vi "PumpValveHeater2.vi"() -> ()   [LabVIEW 2015]
uses:
  PumpValve.ctl
  <vilib>/DAQmx/read.llb/DAQmx Read (Analog 1D Wfm NChan 1Samp).vi
  <vilib>/DAQmx/write.llb/DAQmx Write (Digital 1D Bool NChan 1Samp 1Line).vi
  <vilib>/DAQmx/miscellaneous.llb/DAQmx Fill In Error Info.vi
  <vilib>/addons/control/pid/pid.llb/PID (DBL).vi
  <vilib>/addons/control/pid/pid.llb/PID Advanced (DBL).vi
  <vilib>/addons/control/pid/NI_PID_pid.lvlib
panel:
  out "Temp Chart 2":waveform(dbl)(graph)
  out "Pressure (mBar) 2":dbl format="%#_13g"
  out "Voltage Reading (Pressure)":dbl format="%#_13g"
  out "Pressure Chart":waveform(dbl)(graph)
  in  "stop":bool
  out "Voltage Reading(Temp)":dbl format="%#_13g"
  out "Temperature (Celcius)":dbl format="%#.1g"
  out "Temp(C)":dbl(slide) scale=-10.0..100.0
  out "Temp Chart":waveform(dbl)(graph)
  out "Duty Cycle from Control Value":dbl
  out "Numeric":dbl
  out "Heater On/off":bool
  out "Control Value (Temp Sensor)":dbl(knob) scale=0.0..100.0
  in  "Stop Maintaining Temp":bool
  in  "PID gains Temp":T1={"proportional gain (Kc)"=1.0, "integral time (Ti, min)"=0.01, "derivative time (Td, min)"=0.0} {"derivative time (Td, min)" format="%.3f"; "integral time (Ti, min)" format="%.3f"; "proportional gain (Kc)" format="%.3f"}
  in  "Temp Setting":dbl
  in  "Maintain Temp":bool
  in  "Stop Maintaining Pressure":bool
  in  "PID gains":T1={"proportional gain (Kc)"=1.0, "integral time (Ti, min)"=0.01, "derivative time (Td, min)"=0.0} {"derivative time (Td, min)" format="%.3f"; "integral time (Ti, min)" format="%.3f"; "proportional gain (Kc)" format="%.3f"}
  out "Meter (Pressure Sensor)":dbl(knob) scale=0.0..10.0
  in  "Pressure Setting":dbl
  in  "Maintain pressure":bool
  in  "On/Off Temp":bool
  in  "Manual Mode Temp":bool
  in  "stop controller":bool
  in  "Duty cycle % (0-100) (manual only)":dbl=50.0
  in  "stop PWM":bool
  in  "Steps in a cycle":i32=256
  in  "Cycle time (s)":dbl=5.0
  in  "On/Off (Pump)":bool
  in  "Open/Close (Blue)":bool
  in  "Open/Close (Green)":bool
  in  "Manual Mode Pump/Valve":bool
  out "Invalid fill%":bool
  out "Tank":u32(slide) scale=0.0..100.0
  in  "Drain %":u32
  in  "Fill %":u32
  in  "Drain":bool
  in  "Stop Program":bool
  in  "Fill":bool
  # "Temp only adjusts up (do nothing to cool?)"
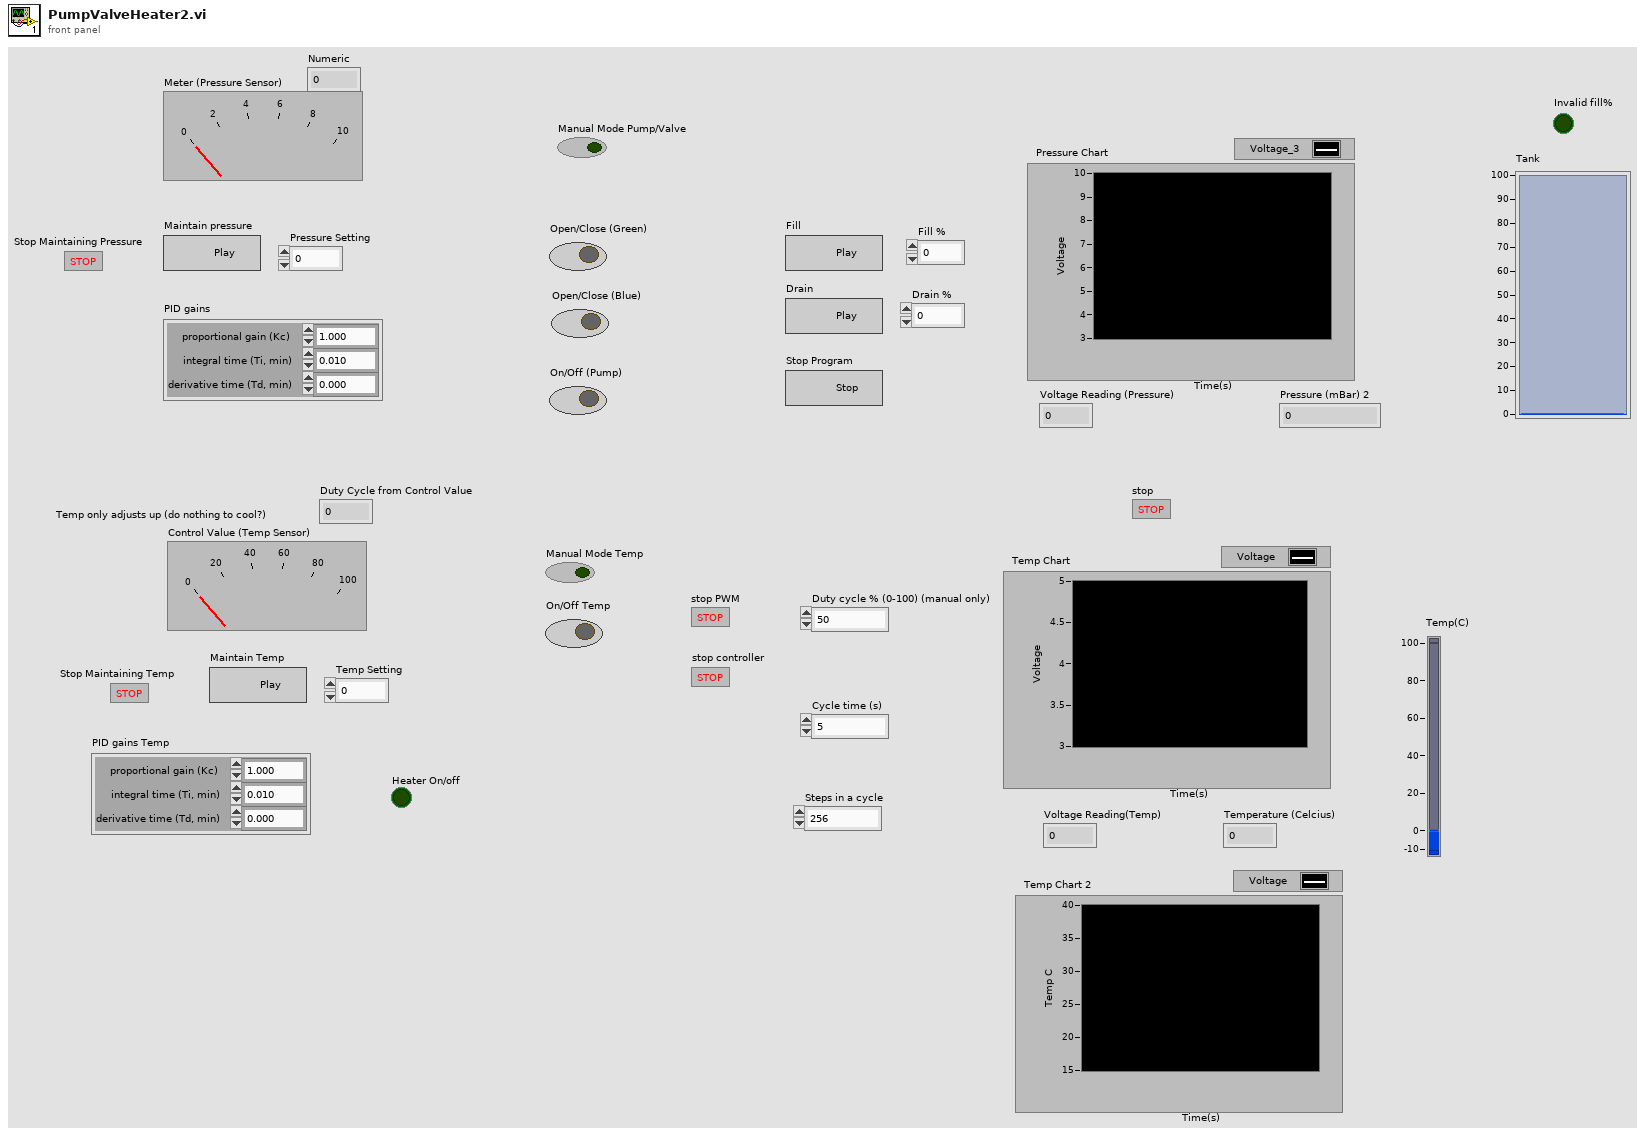
[diagram p1: front panel]
types:
  T1 = cluster{"proportional gain (Kc)":dbl, "integral time (Ti, min)":dbl, "derivative time (Td, min)":dbl}
  T2 = typedef "PumpValve.ctl" = enum16{"PressureSetting", "ManualPressure", "ManualTemp", "Idle Temp", "Set Temp", "Initialize", "Idle", "Fill", "Drain", "Stop"}
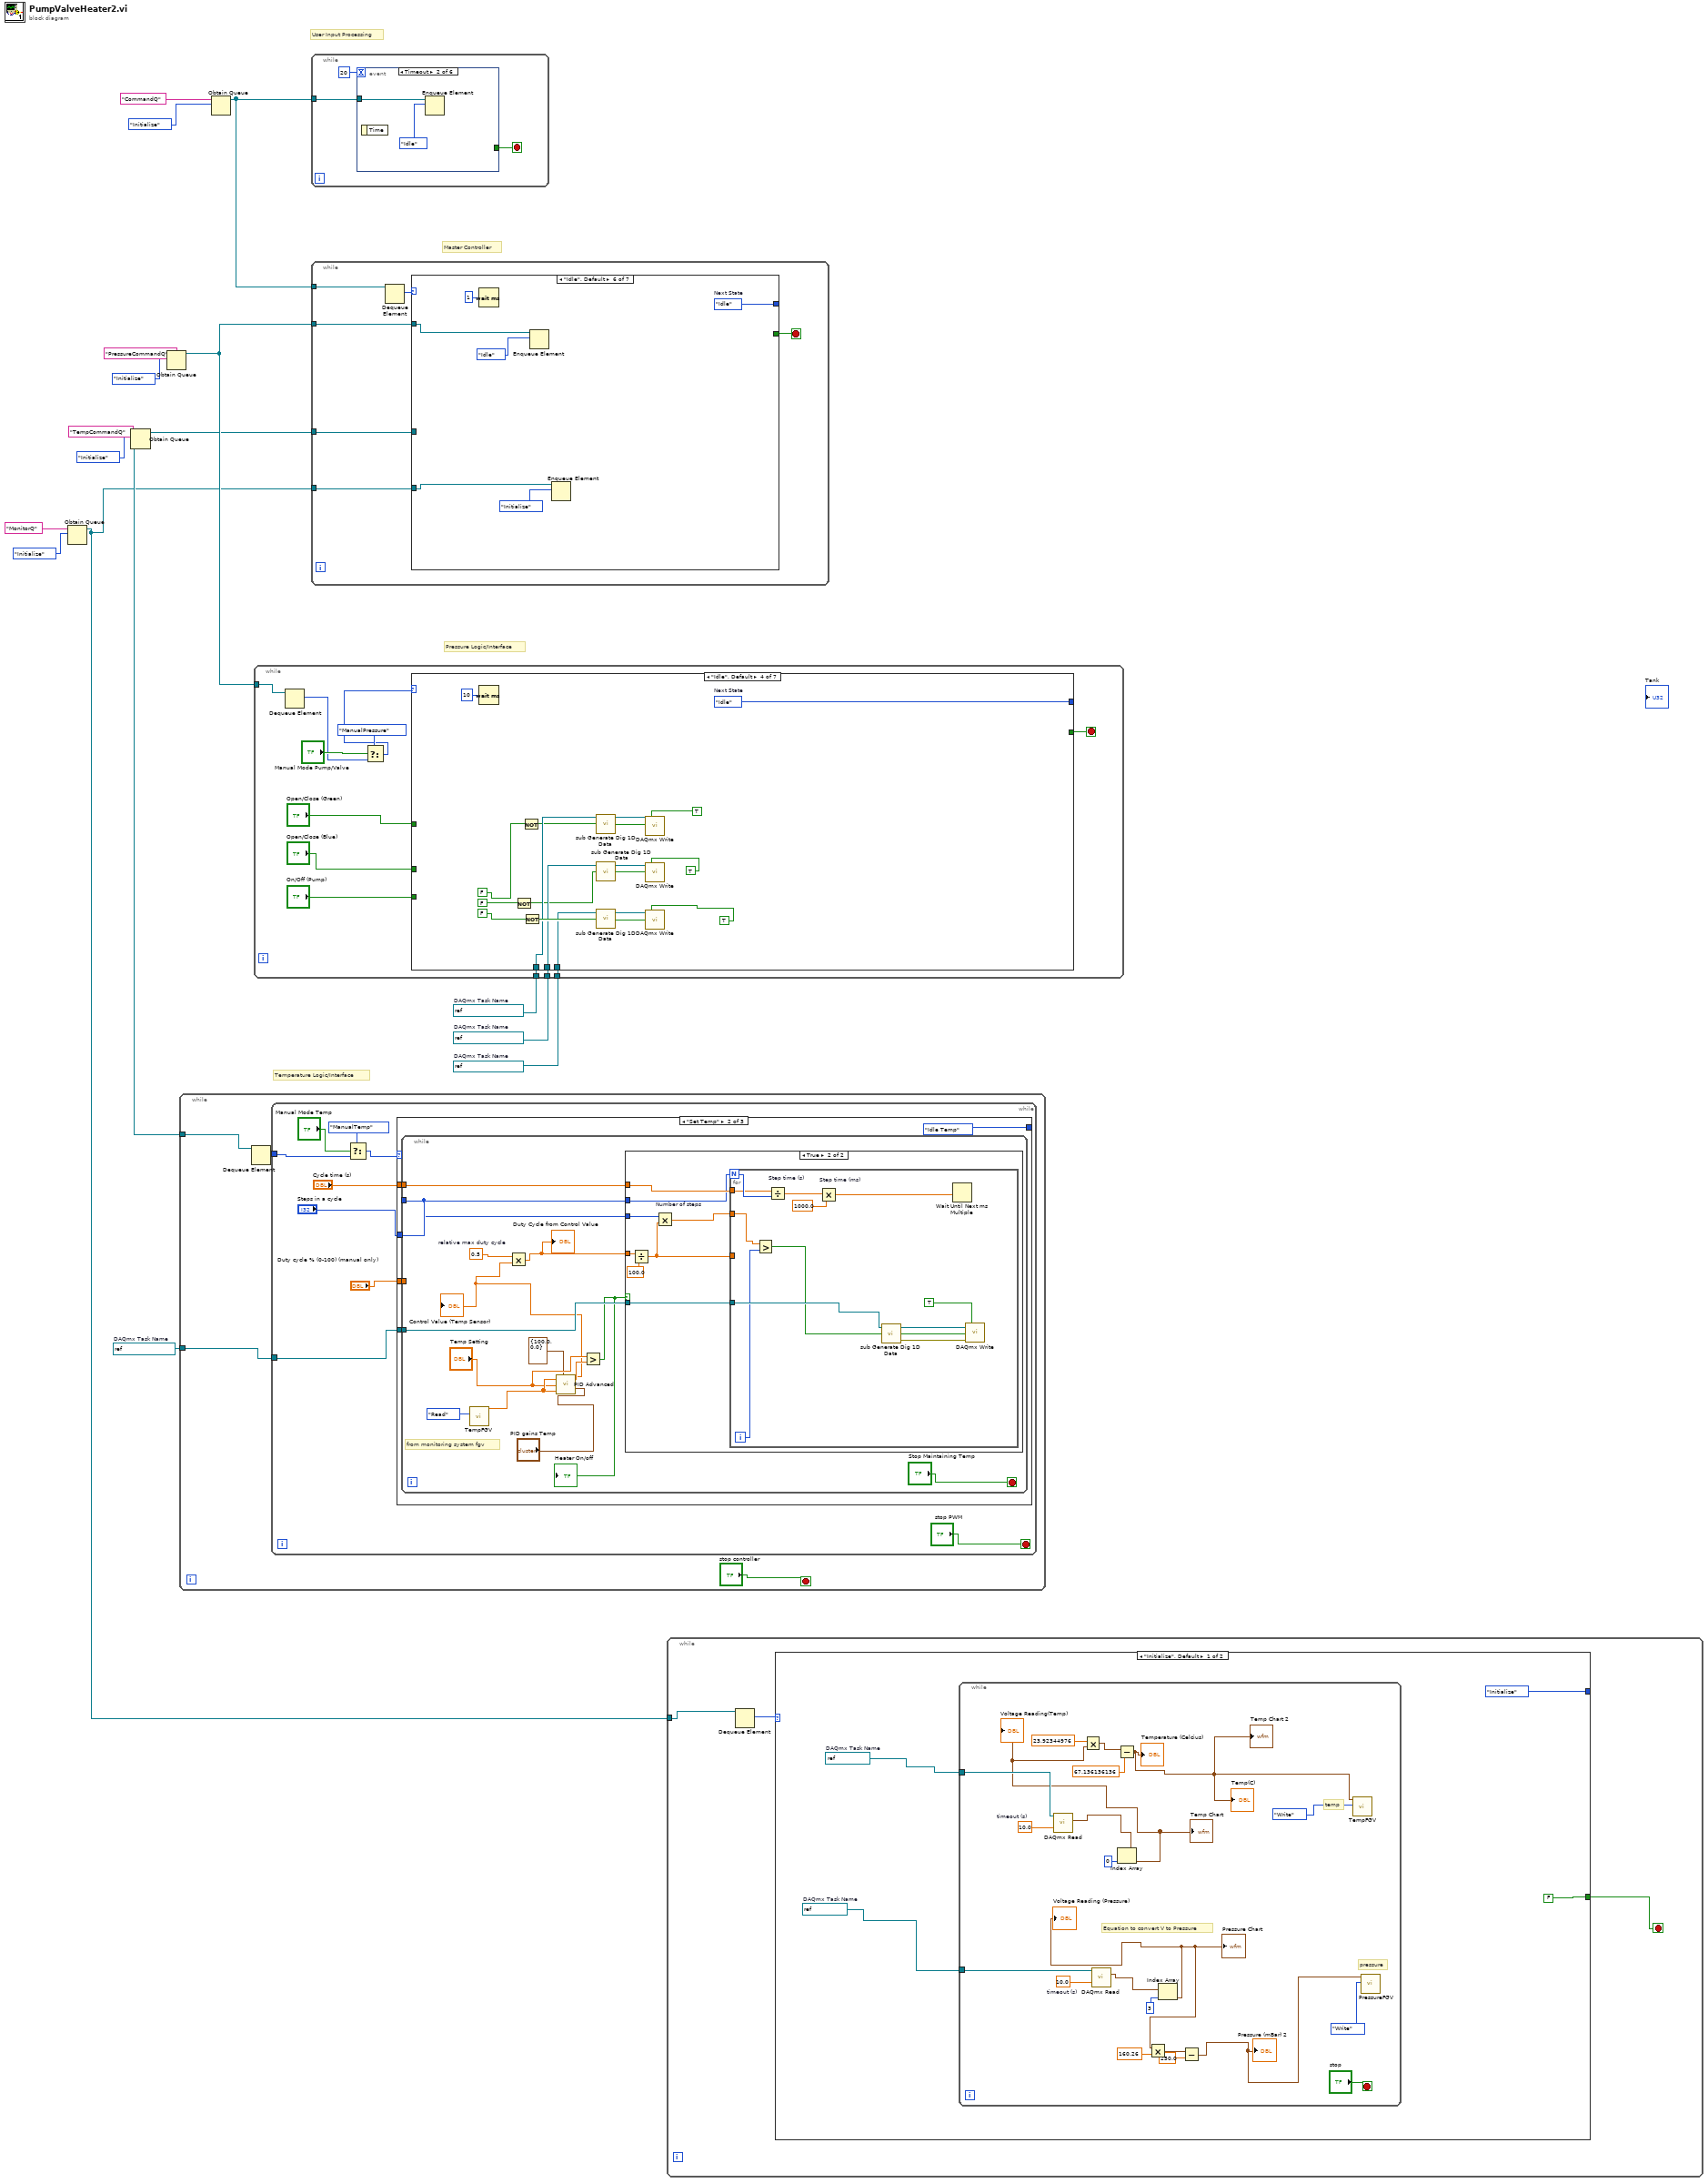
[diagram p0: block diagram]
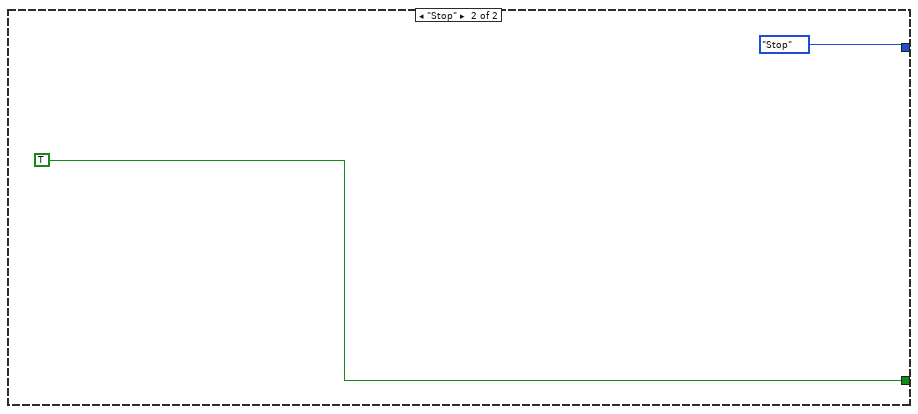
[diagram p2: hidden frame]
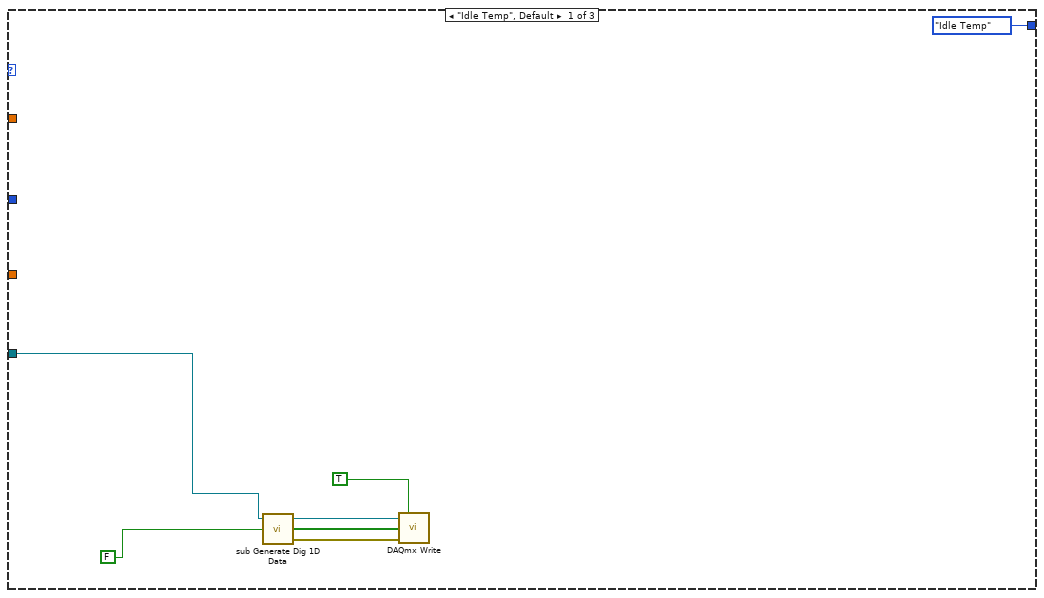
[diagram p3: hidden frame]
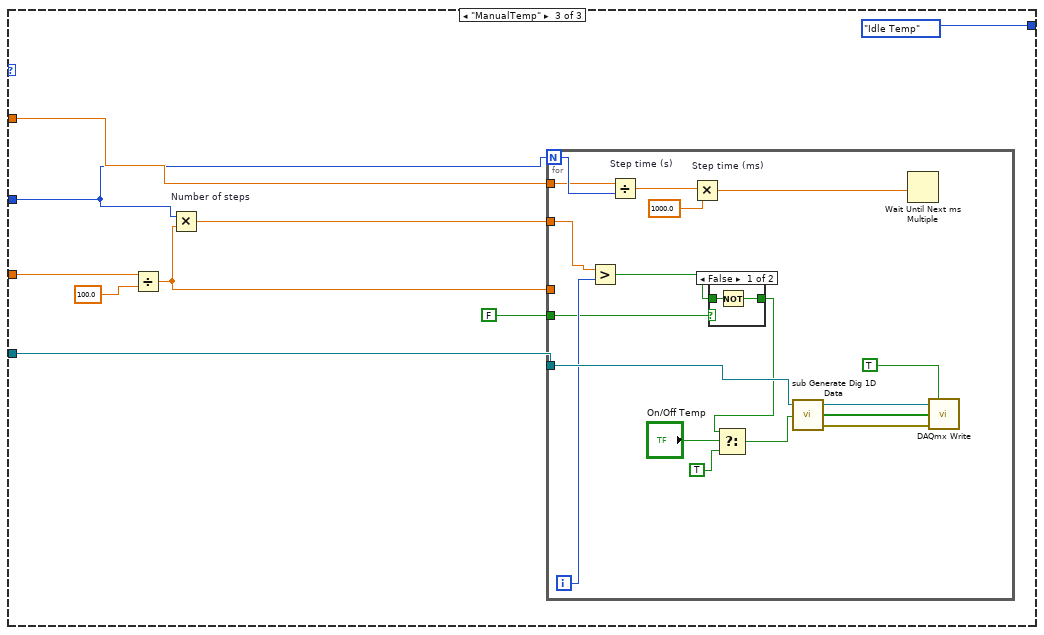
[diagram p5: hidden frame]
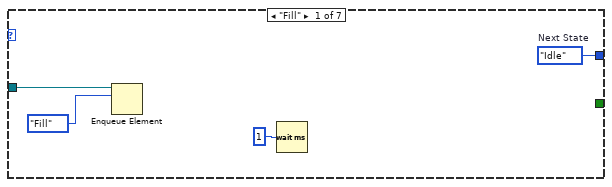
[diagram p7: hidden frame]
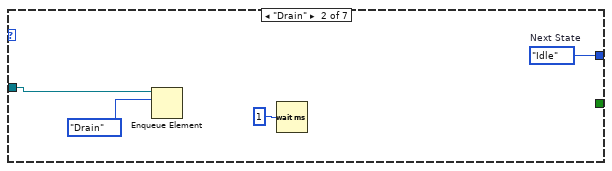
[diagram p8: hidden frame]
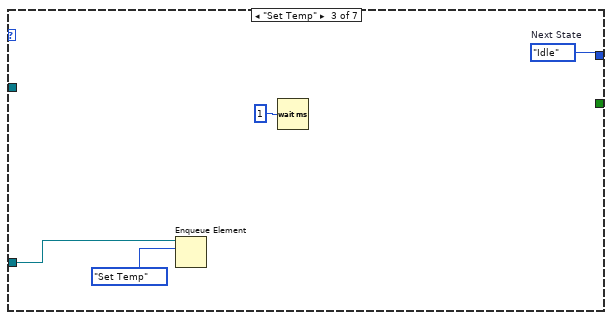
[diagram p9: hidden frame]
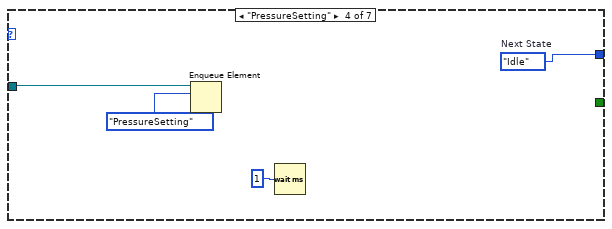
[diagram p10: hidden frame]
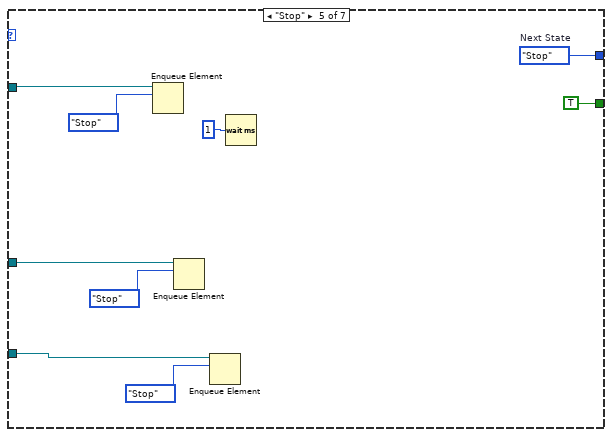
[diagram p11: hidden frame]
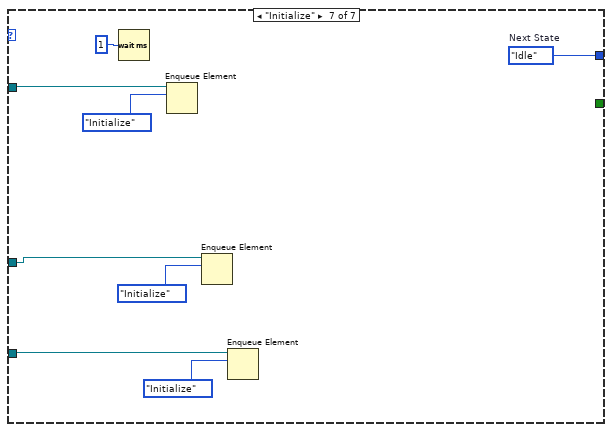
[diagram p12: hidden frame]
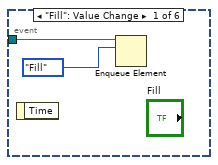
[diagram p13: hidden frame]
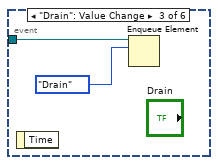
[diagram p14: hidden frame]
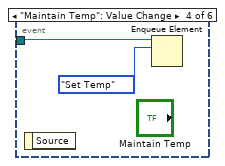
[diagram p15: hidden frame]
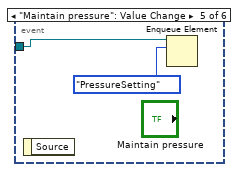
[diagram p16: hidden frame]
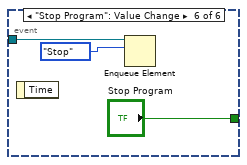
[diagram p17: hidden frame]
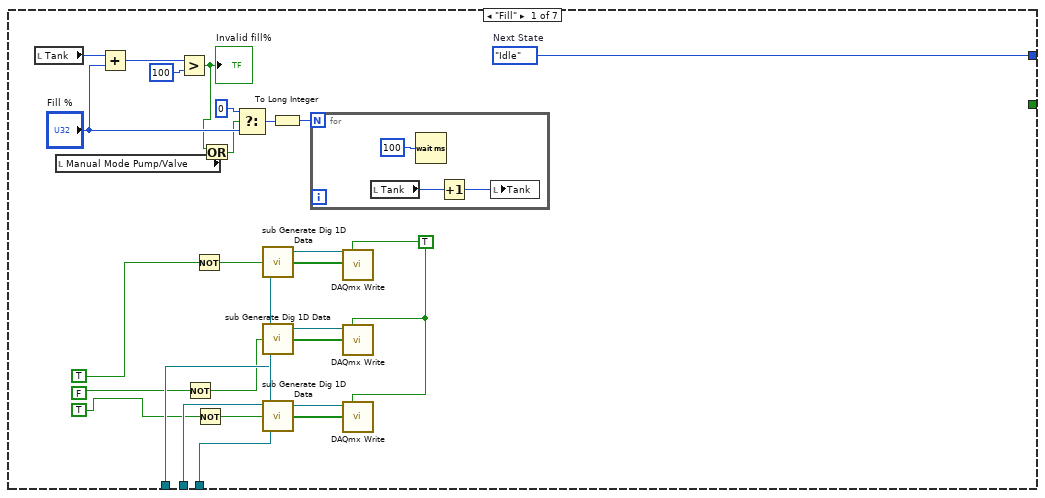
[diagram p18: hidden frame]
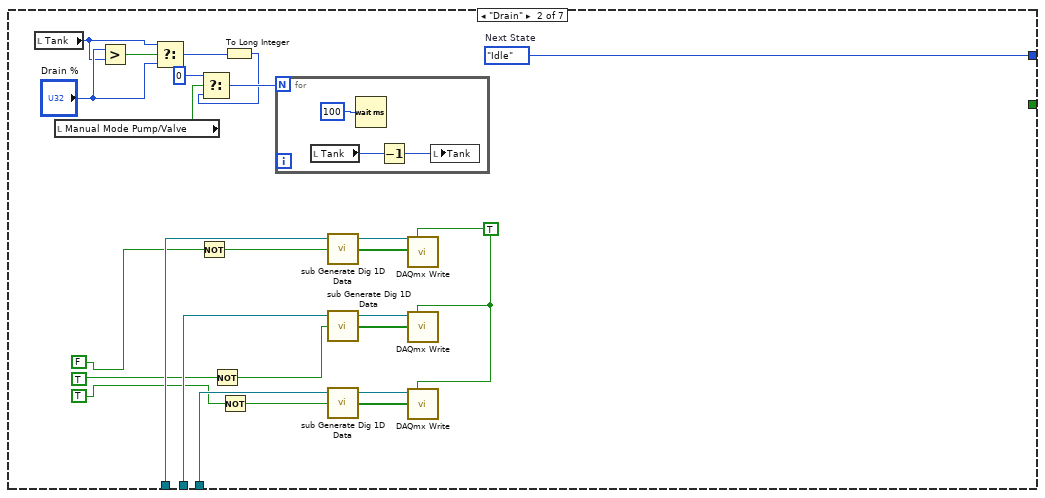
[diagram p19: hidden frame]
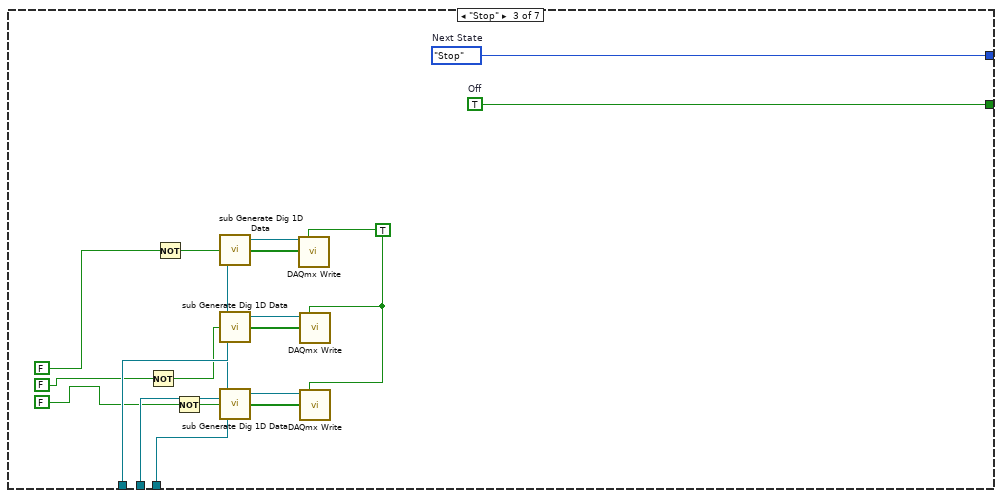
[diagram p20: hidden frame]
diagram:
  w7 = refnum<k21> "P0L0DigitalOut"  # DAQmx Task Name
  w12 = refnum<k21> "DigitalOutGreen"  # DAQmx Task Name
  w13 = refnum<k21> "DigitalOutGreen"  # DAQmx Task Name
  w14 = refnum<k21> "DigitalOutGreen"  # DAQmx Task Name
  # "Temperature Logic/Interface"
  # "Pressure Logic/Interface"
  # "Master Controller"
  # "User Input Processing"
  n1 = Obtain Queue(name (unnamed)="MonitorQ", element data type=PumpValve."Initialize" ("States")) -> (queue out=w1:refnum<queue>)  [unwired: 3 in, 2 out]
  n2 = Obtain Queue(name (unnamed)="TempCommandQ", element data type=PumpValve."Initialize" ("States")) -> (queue out=w4:refnum<queue>)  [unwired: 3 in, 2 out]
  n3 = Obtain Queue(name (unnamed)="PressureCommandQ", element data type=PumpValve."Initialize" ("States")) -> (queue out=w8:refnum<queue>)  [unwired: 3 in, 2 out]
  n4 = while {
    tunnel: w7 -> [w20]
    tunnel: w4 -> [w19]
    stop <- "stop controller" stop-if-true
    n5 = Dequeue Element(queue=w19) -> (element=w18:T2)  [unwired: 2 in, 3 out]
    n6 = while {
      tunnel: w20 -> [w29]
      tunnel: w18 -> [w24]
      stop <- "stop PWM" stop-if-true
      n7 = Select(t=PumpValve."ManualTemp", s="Manual Mode Temp", f=w24) -> (s? t:f=w23:T2)
      n8 = case shown="\"Set Temp\"" w23 {
        tunnel: w29 -> [w31 w41 w83]
        tunnel: [PumpValve."Idle Temp" ("States") PumpValve."Idle Temp" ("States") PumpValve."Idle Temp" ("States")] -> _
        tunnel: "Cycle time (s)" -> [_ w39 w77]
        tunnel: "Steps in a cycle" -> [_ w38 w76]
        tunnel: "Duty cycle % (0-100) (manual only)" -> [_ w37 w75]
        frame "Idle Temp", Default {
          n9 = call <vilib>:"sub Generate Dig 1D Data.vi"("initial value"=FALSE, "task in"=w31) -> ("error out"=w33:errorcluster, "Data"=w34:bool[], "task out"=w35:refnum<k21>)  [unwired: 1 in]
          n10 = call-poly <vilib>:"DAQmx Write.vi"("task/channels in"=w35, "auto start"=TRUE, "data"=w34, "error in"=w33) -> ()  [unwired: 9 in, 3 out]
        }
        frame "Set Temp" {
          n11 = while {
            tunnel: w41 -> [w54]
            tunnel: w39 -> [w53]
            tunnel: w38 -> [w51]
            tunnel: w37 -> [_]
            stop <- "Stop Maintaining Temp" stop-if-true
            w42 = 0.5  # relative max duty cycle
            # "from monitoring system fgv"
            n12 = call "TempFGV.vi"("Command"=enum16{"Write", "Read"}."Read") -> ("OUT"=w46:dbl)  [unwired: 10 in]
            n13 = call-poly <vilib>:"PID Advanced.vi"("setpoint"="Temp Setting", "output range"=cluster{"output high":dbl, "output low":dbl} {"output high"=100.0, "output low"=0.0}, "process variable"=w46, "PID gains"="PID gains Temp") -> ("output"=w44:dbl)  [unwired: 10 in, 1 out]
            "Control Value (Temp Sensor)" <- w44
            n14 = Multiply(x=w42, y=w44) -> (x*y=w48:dbl)
            "Duty Cycle from Control Value" <- w48
            n15 = Greater?(x="Temp Setting", y=w46) -> (0:w50:bool)
            "Heater On/off" <- w50
            n16 = case shown="True" w50 {
              tunnel: w54 -> [_ w61]
              tunnel: w53 -> [_ w57]
              tunnel: w51 -> [_ w56]
              tunnel: w48 -> [_ w55]
              tunnel: w51 -> [_ _]
              frame False {
              }
              frame True {
                n17 = Divide(x=w55, y=100.0) -> (x/y=w59:dbl)
                n18 = Multiply "Number of steps"(x=w56, y=w59) -> (x*y=w58:dbl)
                n19 = for {
                  N: w56 -> [w70]
                  tunnel: w61 -> [w71]
                  tunnel: w59 -> [_]
                  tunnel: w57 -> [w69]
                  tunnel: w58 -> [w65]
                  i -> [w64]
                  n20 = Greater?(x=w65, y=w64) -> (0:w62:bool)
                  n21 = Divide "Step time (s)"(x=w69, y=w70) -> (x/y=w68:dbl)
                  n22 = Multiply "Step time (ms)"(x=w68, y=1000.0) -> (x*y=w66:dbl)
                  n23 = call <vilib>:"sub Generate Dig 1D Data.vi"("initial value"=w62, "task in"=w71) -> ("error out"=w73:errorcluster, "Data"=w63:bool[], "task out"=w72:refnum<k21>)  [unwired: 1 in]
                  n24 = Wait Until Next ms Multiple(millisecond multiple=w66) -> ()  [unwired: 1 out]
                  n25 = call-poly <vilib>:"DAQmx Write.vi"("task/channels in"=w72, "auto start"=TRUE, "data"=w63, "error in"=w73) -> ()  [unwired: 9 in, 3 out]
                }
              }
            }
          }
        }
        frame "ManualTemp" {
          n26 = Divide(x=w75, y=100.0) -> (x/y=w81:dbl)
          n27 = Multiply "Number of steps"(x=w76, y=w81) -> (x*y=w80:dbl)
          n28 = for {
            N: w76 -> [w96]
            tunnel: w83 -> [w97]
            tunnel: w81 -> [_]
            tunnel: w77 -> [w95]
            tunnel: w80 -> [w91]
            tunnel: FALSE -> [w88]
            i -> [w90]
            n29 = Greater?(x=w91, y=w90) -> (0:w89:bool)
            n30 = Divide "Step time (s)"(x=w95, y=w96) -> (x/y=w94:dbl)
            n31 = Multiply "Step time (ms)"(x=w94, y=1000.0) -> (x*y=w92:dbl)
            n32 = case shown="False" w88 {
              tunnel: [w102 w104] -> w86
              tunnel: w89 -> [w103 w104]
              frame False {
                n33 = Not(x=w103) -> (.not. x?=w102:bool)
              }
              frame True {
              }
            }
            n34 = Select(t=w86, s="On/Off Temp", f=TRUE) -> (s? t:f=w85:bool)
            n35 = call <vilib>:"sub Generate Dig 1D Data.vi"("initial value"=w85, "task in"=w97) -> ("error out"=w100:errorcluster, "Data"=w99:bool[], "task out"=w98:refnum<k21>)  [unwired: 1 in]
            n36 = Wait Until Next ms Multiple(millisecond multiple=w92) -> ()  [unwired: 1 out]
            n37 = call-poly <vilib>:"DAQmx Write.vi"("task/channels in"=w98, "auto start"=TRUE, "data"=w99, "error in"=w100) -> ()  [unwired: 9 in, 3 out]
          }
        }
      }
    }
  }
  n38 = Obtain Queue(name (unnamed)="CommandQ", element data type=PumpValve."Initialize" ("States")) -> (queue out=w11:refnum<queue>)  [unwired: 3 in, 2 out]
  n39 = while {
    tunnel: w8 -> [w116]
    tunnel: w14 -> [w112]
    tunnel: w13 -> [w113]
    tunnel: w12 -> [w114]
    stop <- w115 stop-if-true
    n40 = Dequeue Element(queue=w116) -> (element=w109:T2)  [unwired: 2 in, 3 out]
    n41 = Select(t=PumpValve."ManualPressure", s="Manual Mode Pump/Valve", f=w109) -> (s? t:f=w108:T2)
    n42 = case shown="\"Idle\", Default" w108 {
      tunnel: [w143 w171 w192 w212 w232 w236 w279] -> _
      tunnel: [_ _ w178 _ _ _ _] -> w115
      tunnel: w114 -> [w125 w153 w182 w200 w220 w233 w268]
      tunnel: w113 -> [w124 w154 w183 w199 w219 w234 w269]
      tunnel: w112 -> [w123 w155 w184 w198 w218 w235 w270]
      tunnel: "Open/Close (Green)" -> [_ _ _ _ w215 _ _]
      tunnel: "Open/Close (Blue)" -> [_ _ _ _ w214 _ _]
      tunnel: "On/Off (Pump)" -> [_ _ _ _ w213 _ _]
      frame "Fill" {
        w132 = TRUE
        w143 = PumpValve."Idle"  # Next State
        n43 = local read "Tank"() -> (w142:u32)
        n44 = local read "Manual Mode Pump/Valve"() -> (w134:bool)
        n45 = Add(x=w142, y="Fill %") -> (x+y=w140:u32)
        n46 = Greater?(x=w140, y=u32 100) -> (0:w135:bool)
        "Invalid fill%" <- w135
        n47 = Not(x=FALSE) -> (.not. x?=w120:bool)
        n48 = Not(x=TRUE) -> (.not. x?=w121:bool)
        n49 = Not(x=TRUE) -> (.not. x?=w122:bool)
        n50 = Or(x=w135, y=w134) -> (x .or. y?=w133:bool)
        n51 = Select(t=u32 0, s=w133, f="Fill %") -> (s? t:f=w137:u32)
        n52 = call <vilib>:"sub Generate Dig 1D Data.vi"("initial value"=w121, "task in"=w123) -> ("Data"=w127:bool[], "task out"=w131:refnum<k21>)  [unwired: 1 in, 1 out]
        n53 = call <vilib>:"sub Generate Dig 1D Data.vi"("initial value"=w120, "task in"=w124) -> ("Data"=w128:bool[], "task out"=w130:refnum<k21>)  [unwired: 1 in, 1 out]
        n54 = call <vilib>:"sub Generate Dig 1D Data.vi"("initial value"=w122, "task in"=w125) -> ("Data"=w126:bool[], "task out"=w129:refnum<k21>)  [unwired: 1 in, 1 out]
        n55 = To Long Integer(number=w137) -> (32bit integer=w136:i32)
        n56 = for {
          N: w136 -> [_]
          n57 = local read "Tank"() -> (w146:u32)
          n58 = Wait (ms)(milliseconds to wait=u32 100 ("y")) -> ()  [unwired: 1 out]
          n59 = Increment(x=w146) -> (x+1=w145:u32)
          n60 = local write "Tank"(w145) -> ()
        }
        n61 = call-poly <vilib>:"DAQmx Write.vi"("task/channels in"=w131, "auto start"=w132, "data"=w127) -> ()  [unwired: 10 in, 3 out]
        n62 = call-poly <vilib>:"DAQmx Write.vi"("task/channels in"=w130, "auto start"=w132, "data"=w128) -> ()  [unwired: 10 in, 3 out]
        n63 = call-poly <vilib>:"DAQmx Write.vi"("task/channels in"=w129, "auto start"=w132, "data"=w126) -> ()  [unwired: 10 in, 3 out]
      }
      frame "Drain" {
        w156 = TRUE
        w171 = PumpValve."Idle"  # Next State
        n64 = local read "Tank"() -> (w168:u32)
        n65 = local read "Manual Mode Pump/Valve"() -> (w166:bool)
        n66 = Greater?(x="Drain %", y=w168) -> (0:w167:bool)
        n67 = Select(t=w168, s=w167, f="Drain %") -> (s? t:f=w170:u32)
        n68 = Not(x=FALSE) -> (.not. x?=w151:bool)
        n69 = Not(x=TRUE) -> (.not. x?=w150:bool)
        n70 = Not(x=TRUE) -> (.not. x?=w152:bool)
        n71 = To Long Integer(number=w170) -> (32bit integer=w163:i32)
        n72 = Select(t=0, s=w166, f=w163) -> (s? t:f=w164:i32)
        n73 = for {
          N: w164 -> [_]
          n74 = local read "Tank"() -> (w173:u32)
          n75 = Wait (ms)(milliseconds to wait=u32 100) -> ()  [unwired: 1 out]
          n76 = Decrement(x=w173) -> (x-1=w174:u32)
          n77 = local write "Tank"(w174) -> ()
        }
        n78 = call <vilib>:"sub Generate Dig 1D Data.vi"("initial value"=w151, "task in"=w155) -> ("Data"=w161:bool[], "task out"=w157:refnum<k21>)  [unwired: 1 in, 1 out]
        n79 = call <vilib>:"sub Generate Dig 1D Data.vi"("initial value"=w150, "task in"=w154) -> ("Data"=w160:bool[], "task out"=w158:refnum<k21>)  [unwired: 1 in, 1 out]
        n80 = call <vilib>:"sub Generate Dig 1D Data.vi"("initial value"=w152, "task in"=w153) -> ("Data"=w162:bool[], "task out"=w159:refnum<k21>)  [unwired: 1 in, 1 out]
        n81 = call-poly <vilib>:"DAQmx Write.vi"("task/channels in"=w157, "auto start"=w156, "data"=w161) -> ()  [unwired: 10 in, 3 out]
        n82 = call-poly <vilib>:"DAQmx Write.vi"("task/channels in"=w158, "auto start"=w156, "data"=w160) -> ()  [unwired: 10 in, 3 out]
        n83 = call-poly <vilib>:"DAQmx Write.vi"("task/channels in"=w159, "auto start"=w156, "data"=w162) -> ()  [unwired: 10 in, 3 out]
      }
      frame "Stop" {
        w191 = TRUE
        w178 = TRUE  # Off
        w192 = PumpValve."Stop"  # Next State
        n84 = Not(x=FALSE) -> (.not. x?=w179:bool)
        n85 = Not(x=FALSE) -> (.not. x?=w180:bool)
        n86 = Not(x=FALSE) -> (.not. x?=w181:bool)
        n87 = call <vilib>:"sub Generate Dig 1D Data.vi"("initial value"=w180, "task in"=w184) -> ("Data"=w186:bool[], "task out"=w190:refnum<k21>)  [unwired: 1 in, 1 out]
        n88 = call <vilib>:"sub Generate Dig 1D Data.vi"("initial value"=w179, "task in"=w183) -> ("Data"=w187:bool[], "task out"=w189:refnum<k21>)  [unwired: 1 in, 1 out]
        n89 = call <vilib>:"sub Generate Dig 1D Data.vi"("initial value"=w181, "task in"=w182) -> ("Data"=w185:bool[], "task out"=w188:refnum<k21>)  [unwired: 1 in, 1 out]
        n90 = call-poly <vilib>:"DAQmx Write.vi"("task/channels in"=w190, "auto start"=w191, "data"=w186) -> ()  [unwired: 10 in, 3 out]
        n91 = call-poly <vilib>:"DAQmx Write.vi"("task/channels in"=w189, "auto start"=w191, "data"=w187) -> ()  [unwired: 10 in, 3 out]
        n92 = call-poly <vilib>:"DAQmx Write.vi"("task/channels in"=w188, "auto start"=w191, "data"=w185) -> ()  [unwired: 10 in, 3 out]
      }
      frame "Idle", Default {
        w212 = PumpValve."Idle"  # Next State
        n93 = Wait (ms)(milliseconds to wait=u32 10) -> ()  [unwired: 1 out]
        n94 = Not(x=FALSE) -> (.not. x?=w196:bool)
        n95 = Not(x=FALSE) -> (.not. x?=w197:bool)
        n96 = Not(x=FALSE) -> (.not. x?=w203:bool)
        n97 = call <vilib>:"sub Generate Dig 1D Data.vi"("initial value"=w197, "task in"=w198) -> ("Data"=w205:bool[], "task out"=w209:refnum<k21>)  [unwired: 1 in, 1 out]
        n98 = call <vilib>:"sub Generate Dig 1D Data.vi"("initial value"=w196, "task in"=w199) -> ("Data"=w206:bool[], "task out"=w208:refnum<k21>)  [unwired: 1 in, 1 out]
        n99 = call <vilib>:"sub Generate Dig 1D Data.vi"("initial value"=w203, "task in"=w200) -> ("Data"=w204:bool[], "task out"=w207:refnum<k21>)  [unwired: 1 in, 1 out]
        n100 = call-poly <vilib>:"DAQmx Write.vi"("task/channels in"=w209, "auto start"=TRUE, "data"=w205) -> ()  [unwired: 10 in, 3 out]
        n101 = call-poly <vilib>:"DAQmx Write.vi"("task/channels in"=w208, "auto start"=TRUE, "data"=w206) -> ()  [unwired: 10 in, 3 out]
        n102 = call-poly <vilib>:"DAQmx Write.vi"("task/channels in"=w207, "auto start"=TRUE, "data"=w204) -> ()  [unwired: 10 in, 3 out]
      }
      frame "ManualPressure" {
        w232 = PumpValve."Idle"  # Next State
        n103 = Wait (ms)(milliseconds to wait=u32 10) -> ()  [unwired: 1 out]
        n104 = Not(x=w214) -> (.not. x?=w216:bool)
        n105 = Not(x=w215) -> (.not. x?=w217:bool)
        n106 = Not(x=w213) -> (.not. x?=w223:bool)
        n107 = call <vilib>:"sub Generate Dig 1D Data.vi"("initial value"=w217, "task in"=w218) -> ("Data"=w225:bool[], "task out"=w229:refnum<k21>)  [unwired: 1 in, 1 out]
        n108 = call <vilib>:"sub Generate Dig 1D Data.vi"("initial value"=w216, "task in"=w219) -> ("Data"=w226:bool[], "task out"=w228:refnum<k21>)  [unwired: 1 in, 1 out]
        n109 = call <vilib>:"sub Generate Dig 1D Data.vi"("initial value"=w223, "task in"=w220) -> ("Data"=w224:bool[], "task out"=w227:refnum<k21>)  [unwired: 1 in, 1 out]
        n110 = call-poly <vilib>:"DAQmx Write.vi"("task/channels in"=w229, "auto start"=TRUE, "data"=w225) -> ()  [unwired: 10 in, 3 out]
        n111 = call-poly <vilib>:"DAQmx Write.vi"("task/channels in"=w228, "auto start"=TRUE, "data"=w226) -> ()  [unwired: 10 in, 3 out]
        n112 = call-poly <vilib>:"DAQmx Write.vi"("task/channels in"=w227, "auto start"=TRUE, "data"=w224) -> ()  [unwired: 10 in, 3 out]
      }
      frame "PressureSetting" {
        w236 = PumpValve."Idle"  # Next State
        n113 = while {
          tunnel: w235 -> [w242]
          tunnel: w234 -> [w241]
          tunnel: w233 -> [w240]
          stop <- "Stop Maintaining Pressure" stop-if-true
          # "from monitoring system"
          # "output to hardware"
          n114 = call "PressureFGV.vi"("IN"=enum16{"Write", "Read"}."Read" ("Command")) -> ("OUT"=w256:dbl)  [unwired: 10 in]
          n115 = call-poly <vilib>:"PID.vi"("PID gains"="PID gains", "process variable"=w256, "setpoint"="Pressure Setting") -> ("output"=w239:dbl)  [unwired: 7 in, 1 out]
          "Meter (Pressure Sensor)" <- w239
          "Numeric" <- w239
          n116 = Greater?(x=w239, y=0.0) -> (0:w237:bool)
          n117 = Not(x=w237) -> (.not. x?=w254:bool)
          n118 = Not(x=w237) -> (.not. x?=w253:bool)
          n119 = Not(x=w237) -> (.not. x?=w250:bool)
          n120 = call <vilib>:"sub Generate Dig 1D Data.vi"("initial value"=w253, "task in"=w242) -> ("Data"=w248:bool[], "task out"=w244:refnum<k21>)  [unwired: 1 in, 1 out]
          n121 = call <vilib>:"sub Generate Dig 1D Data.vi"("initial value"=w254, "task in"=w241) -> ("Data"=w247:bool[], "task out"=w245:refnum<k21>)  [unwired: 1 in, 1 out]
          n122 = call <vilib>:"sub Generate Dig 1D Data.vi"("initial value"=w250, "task in"=w240) -> ("Data"=w249:bool[], "task out"=w246:refnum<k21>)  [unwired: 1 in, 1 out]
          n123 = call-poly <vilib>:"DAQmx Write.vi"("task/channels in"=w244, "auto start"=TRUE, "data"=w248) -> ()  [unwired: 10 in, 3 out]
          n124 = call-poly <vilib>:"DAQmx Write.vi"("task/channels in"=w245, "auto start"=TRUE, "data"=w247) -> ()  [unwired: 10 in, 3 out]
          n125 = call-poly <vilib>:"DAQmx Write.vi"("task/channels in"=w246, "auto start"=TRUE, "data"=w249) -> ()  [unwired: 10 in, 3 out]
        }
      }
      frame "Initialize" {
        w279 = PumpValve."Idle"  # Next State
        n126 = Wait (ms)(milliseconds to wait=u32 1) -> ()  [unwired: 1 out]
        n127 = Not(x=FALSE) -> (.not. x?=w264:bool)
        n128 = Not(x=FALSE) -> (.not. x?=w263:bool)
        n129 = Not(x=FALSE) -> (.not. x?=w267:bool)
        n130 = call <vilib>:"sub Generate Dig 1D Data.vi"("initial value"=w264, "task in"=w270) -> ("Data"=w272:bool[], "task out"=w276:refnum<k21>)  [unwired: 1 in, 1 out]
        n131 = call <vilib>:"sub Generate Dig 1D Data.vi"("initial value"=w263, "task in"=w269) -> ("Data"=w273:bool[], "task out"=w275:refnum<k21>)  [unwired: 1 in, 1 out]
        n132 = call <vilib>:"sub Generate Dig 1D Data.vi"("initial value"=w267, "task in"=w268) -> ("Data"=w271:bool[], "task out"=w274:refnum<k21>)  [unwired: 1 in, 1 out]
        n133 = call-poly <vilib>:"DAQmx Write.vi"("task/channels in"=w276, "auto start"=TRUE, "data"=w272) -> ()  [unwired: 10 in, 3 out]
        n134 = call-poly <vilib>:"DAQmx Write.vi"("task/channels in"=w275, "auto start"=TRUE, "data"=w273) -> ()  [unwired: 10 in, 3 out]
        n135 = call-poly <vilib>:"DAQmx Write.vi"("task/channels in"=w274, "auto start"=TRUE, "data"=w271) -> ()  [unwired: 10 in, 3 out]
      }
    }
  }
  n136 = while {
    tunnel: w11 -> [w281]
    stop <- w280 stop-if-true
    n137 = event shown="[1] Timeout" {
      selector: _ -> [_ _ _ _ _ _]
      dyn-events: _ -> [_ _ _ _ _ _]
      timeout: 20 -> [_ _ _ _ _ _]
      tunnel: w281 -> [w284 w286 w288 w289 w292 w295]
      tunnel: [_ _ _ _ _ "Stop Program"] -> w280
      event "Fill": Value Change {
        n138 = event-data() -> ()  [unwired: 1 in, 1 out]
        n139 = Enqueue Element(queue=w284, element=PumpValve."Fill" ("States")) -> ()  [unwired: 2 in, 3 out]
      }
      event Timeout {
        n140 = event-data() -> ()  [unwired: 1 in, 1 out]
        n141 = Enqueue Element(queue=w286, element=PumpValve."Idle" ("States")) -> ()  [unwired: 2 in, 3 out]
      }
      event "Drain": Value Change {
        n142 = event-data() -> ()  [unwired: 1 in, 1 out]
        n143 = Enqueue Element(queue=w288, element=PumpValve."Drain" ("States")) -> ()  [unwired: 2 in, 3 out]
      }
      event "Maintain Temp": Value Change {
        n144 = event-data() -> ()  [unwired: 1 in, 1 out]
        n145 = Enqueue Element(queue=w289, element=PumpValve."Set Temp" ("States")) -> ()  [unwired: 2 in, 3 out]
      }
      event "Maintain pressure": Value Change {
        n146 = event-data() -> ()  [unwired: 1 in, 1 out]
        n147 = Enqueue Element(queue=w292, element=PumpValve."PressureSetting" ("States")) -> ()  [unwired: 2 in, 3 out]
      }
      event "Stop Program": Value Change {
        n148 = event-data() -> ()  [unwired: 1 in, 1 out]
        n149 = Enqueue Element(queue=w295, element=PumpValve."Stop" ("States")) -> ()  [unwired: 2 in, 3 out]
      }
    }
  }
  n150 = while {
    tunnel: w11 -> [w300]
    tunnel: w8 -> [w299]
    tunnel: w4 -> [w297]
    tunnel: w1 -> [w296]
    stop <- w298 stop-if-true
    n151 = Dequeue Element(queue=w300) -> (element=w301:T2)  [unwired: 2 in, 3 out]
    n152 = case shown="\"Idle\", Default" w301 {
      tunnel: [w305 w309 w311 w315 w326 w332 w340] -> _
      tunnel: w299 -> [w302 w306 _ w314 w323 w329 w337]
      tunnel: [_ _ _ _ TRUE _ _] -> w298
      tunnel: w297 -> [_ _ w310 _ w320 _ w334]
      tunnel: w296 -> [_ _ _ _ w318 w327 w333]
      frame "Fill" {
        w305 = PumpValve."Idle"  # Next State
        n153 = Enqueue Element(queue=w302, element=PumpValve."Fill" ("States")) -> ()  [unwired: 2 in, 3 out]
        n154 = Wait (ms)(milliseconds to wait=u32 1) -> ()  [unwired: 1 out]
      }
      frame "Drain" {
        w309 = PumpValve."Idle"  # Next State
        n155 = Enqueue Element(queue=w306, element=PumpValve."Drain" ("States")) -> ()  [unwired: 2 in, 3 out]
        n156 = Wait (ms)(milliseconds to wait=u32 1) -> ()  [unwired: 1 out]
      }
      frame "Set Temp" {
        w311 = PumpValve."Idle"  # Next State
        n157 = Enqueue Element(queue=w310, element=PumpValve."Set Temp" ("States")) -> ()  [unwired: 2 in, 3 out]
        n158 = Wait (ms)(milliseconds to wait=u32 1) -> ()  [unwired: 1 out]
      }
      frame "PressureSetting" {
        w315 = PumpValve."Idle"  # Next State
        n159 = Enqueue Element(queue=w314, element=PumpValve."PressureSetting" ("States")) -> ()  [unwired: 2 in, 3 out]
        n160 = Wait (ms)(milliseconds to wait=u32 1) -> ()  [unwired: 1 out]
      }
      frame "Stop" {
        w326 = PumpValve."Stop"  # Next State
        n161 = Enqueue Element(queue=w323, element=PumpValve."Stop" ("States")) -> ()  [unwired: 2 in, 3 out]
        n162 = Enqueue Element(queue=w320, element=PumpValve."Stop" ("States")) -> ()  [unwired: 2 in, 3 out]
        n163 = Enqueue Element(queue=w318, element=PumpValve."Stop" ("States")) -> ()  [unwired: 2 in, 3 out]
        n164 = Wait (ms)(milliseconds to wait=u32 1) -> ()  [unwired: 1 out]
      }
      frame "Idle", Default {
        w332 = PumpValve."Idle"  # Next State
        n165 = Wait (ms)(milliseconds to wait=u32 1) -> ()  [unwired: 1 out]
        n166 = Enqueue Element(queue=w329, element=PumpValve."Idle" ("States")) -> ()  [unwired: 2 in, 3 out]
        n167 = Enqueue Element(queue=w327, element=PumpValve."Initialize" ("States")) -> ()  [unwired: 2 in, 3 out]
      }
      frame "Initialize" {
        w340 = PumpValve."Idle"  # Next State
        n168 = Wait (ms)(milliseconds to wait=u32 1) -> ()  [unwired: 1 out]
        n169 = Enqueue Element(queue=w337, element=PumpValve."Initialize" ("States")) -> ()  [unwired: 2 in, 3 out]
        n170 = Enqueue Element(queue=w334, element=PumpValve."Initialize" ("States")) -> ()  [unwired: 2 in, 3 out]
        n171 = Enqueue Element(queue=w333, element=PumpValve."Initialize" ("States")) -> ()  [unwired: 2 in, 3 out]
      }
    }
  }
  n172 = while {
    tunnel: w1 -> [w343]
    stop <- w341 stop-if-true
    n173 = Dequeue Element(queue=w343) -> (element=w342:T2)  [unwired: 2 in, 3 out]
    n174 = case shown="\"Initialize\", Default" w342 {
      tunnel: [FALSE TRUE] -> w341
      tunnel: [PumpValve."Initialize" ("States") PumpValve."Stop" ("States")] -> _
      frame "Initialize", Default {
        w344 = refnum<k21> "A0New1"  # DAQmx Task Name
        w345 = refnum<k21> "A0New1"  # DAQmx Task Name
        n175 = while {
          tunnel: w345 -> [w367]
          tunnel: w344 -> [w361]
          stop <- "stop" stop-if-true
          w360 = 10.0  # timeout (s)
          w368 = 10.0  # timeout (s)
          # "Equation to convert V to Pressure"
          # "pressure"
          # "temp"
          n176 = call-poly <vilib>:"DAQmx Read.vi"("task/channels in"=w367, "timeout"=w368) -> ("data"=w357:waveform(dbl)[])  [unwired: 11 in, 2 out]
          n177 = call-poly <vilib>:"DAQmx Read.vi"("task/channels in"=w361, "timeout"=w360) -> ("data"=w354:waveform(dbl)[])  [unwired: 11 in, 2 out]
          n178 = Index Array(array=w357, index=0) -> (element=w356:waveform(dbl))
          "Voltage Reading(Temp)" <- w356
          "Temp Chart" <- w356
          n179 = Multiply(x=23.92344976, y=w356) -> (x*y=w364:waveform(dbl))
          n180 = Subtract(x=w364, y=67.136136136) -> (x-y=w348:waveform(dbl))
          "Temperature (Celcius)" <- w348
          "Temp(C)" <- w348
          "Temp Chart 2" <- w348
          n181 = Index Array(array=w354, index=3) -> (element=w350:waveform(dbl))
          "Pressure Chart" <- w350
          "Voltage Reading (Pressure)" <- w350
          n182 = Multiply(x=w350, y=160.26) -> (x*y=w352:waveform(dbl))
          n183 = Subtract(x=w352, y=250.0) -> (x-y=w349:waveform(dbl))
          "Pressure (mBar) 2" <- w349
          n184 = call "TempFGV.vi"("Command"=enum16{"Write", "Read"}."Write", "IN"=w348) -> ()  [unwired: 9 in, 1 out]
          n185 = call "PressureFGV.vi"("Command"=enum16{"Write", "Read"}."Write", "IN"=w349) -> ()  [unwired: 9 in, 1 out]
        }
      }
      frame "Stop" {
      }
    }
  }
